vi "Motion Profile Generator-Demo.vi"(0 "Max Speed (rotations/sec)":dbl=3.0, 5 "Max Acceleration (rotations/sec^2)":dbl=1.0, 7 "Max Jerk (rotations/sec^3)":dbl=1.0, 9 "Rotations to Travel":dbl=4.0, 11 "Duration MS":dbl=10.0) -> (4 "Position rotations":dbl[](array[numeric]), 6 "velocity rotations/sec":dbl[](array[numeric]), 8 "acceleration rotations/sec^2":dbl[](array[numeric]), 10 "XY Graph":cluster{dbl[], dbl[]}[](graph))   [LabVIEW 2015]
panel:
  out "Final Position":dbl
  # "This VI uses the \"Copioli\" Method of Motion Profiling. For more information read this chief delphi thread: http://www.chiefdelphi.com/forums/showthread.php?t=98358&highlight=motion+profile"
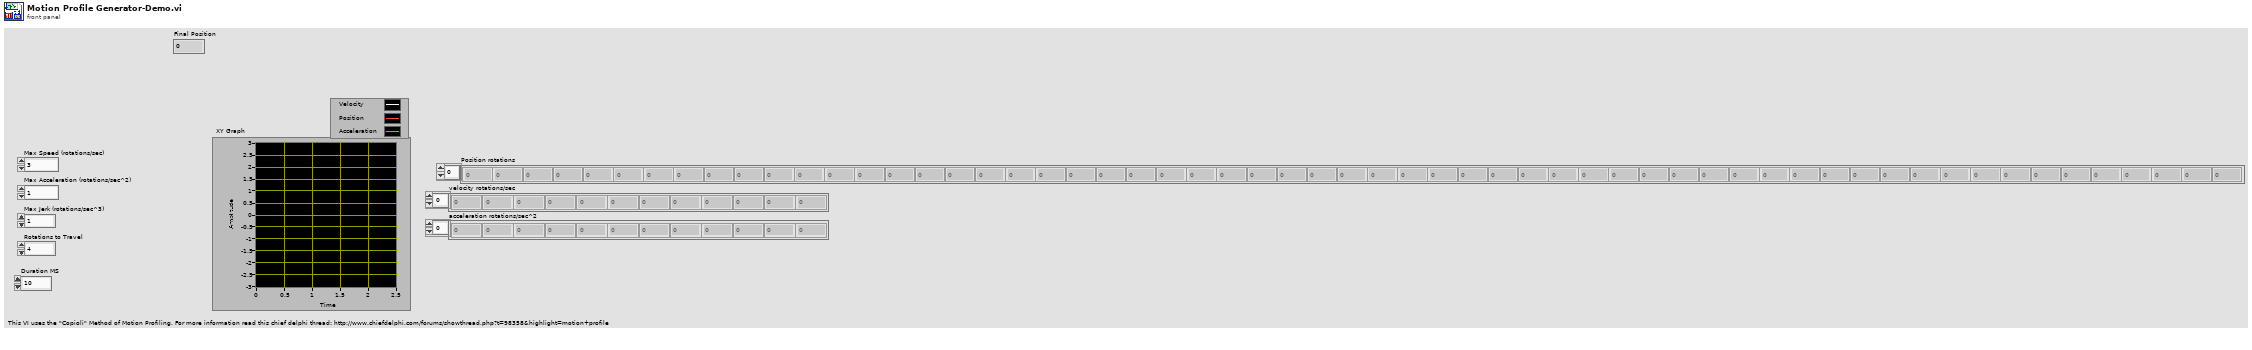
[diagram p1: front panel]
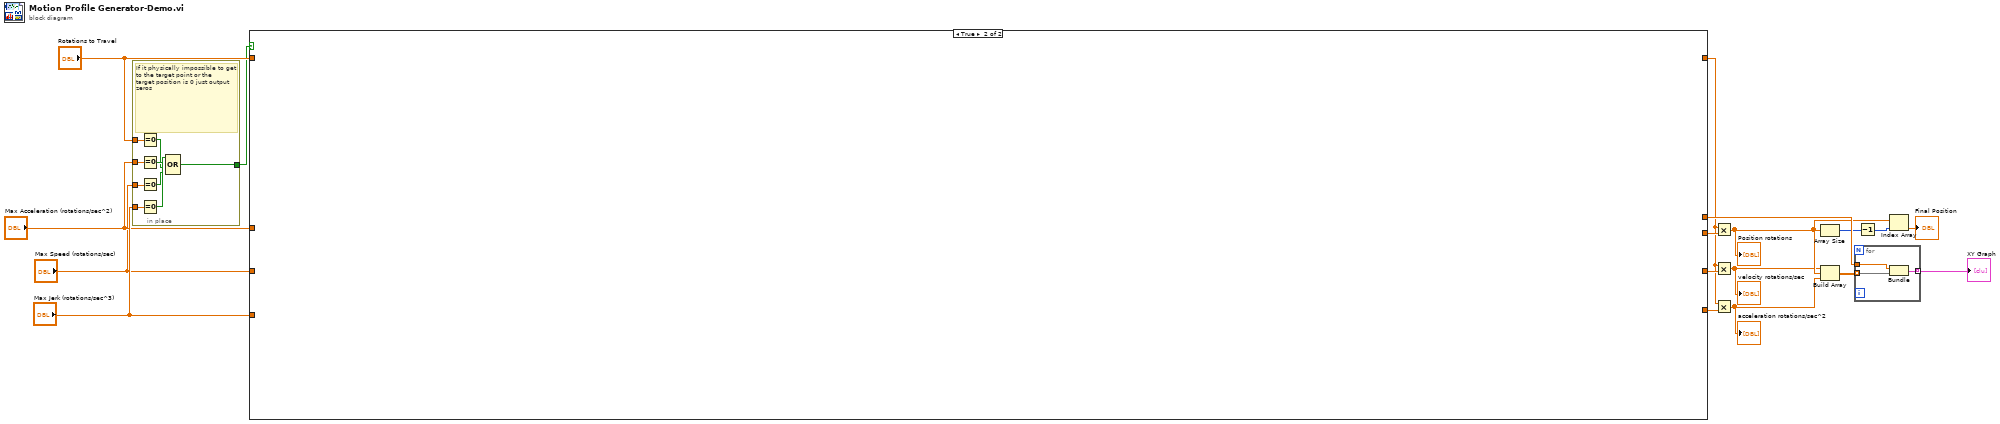
[diagram p0: block diagram]
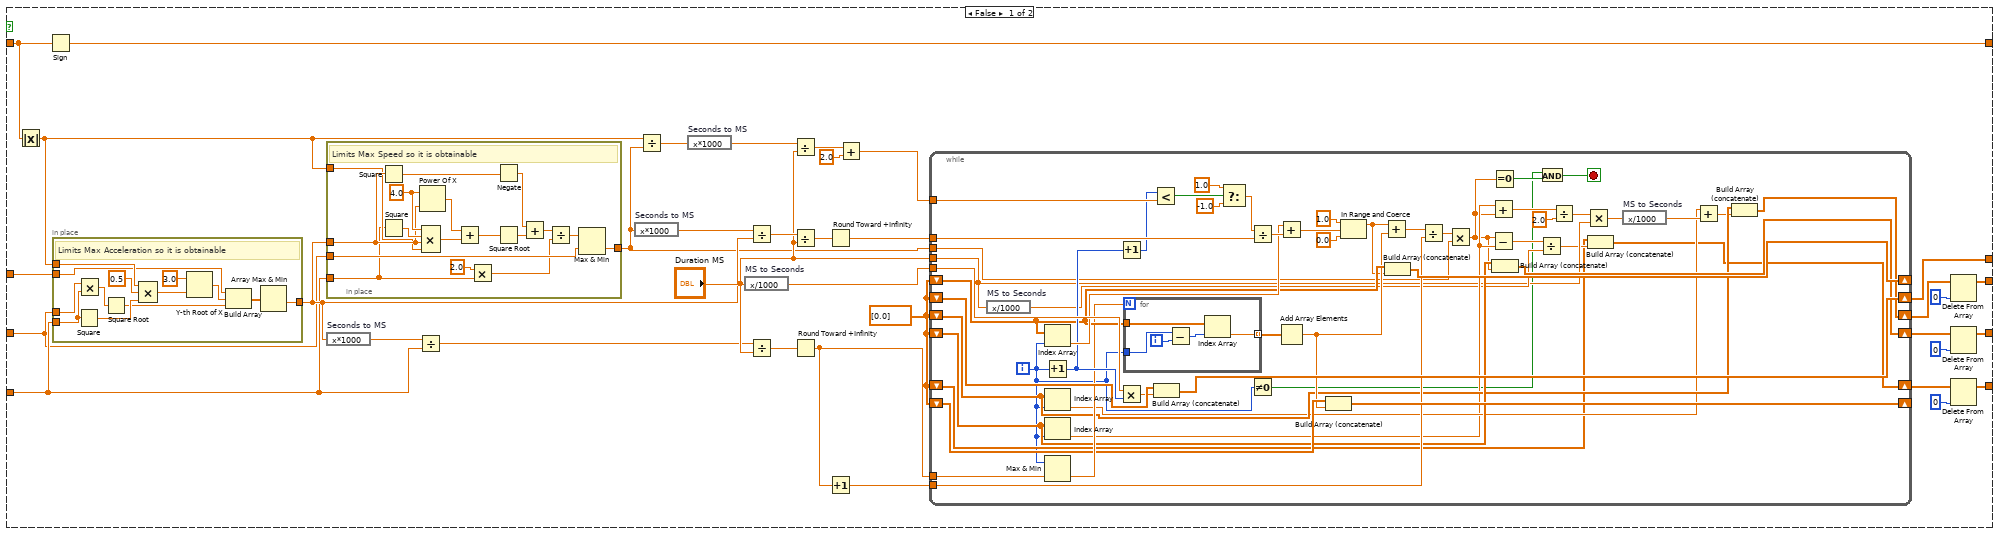
[diagram p2: hidden frame]
diagram:
  n1 = in-place {
    in-place-border: "Max Jerk (rotations/sec^3)" -> [w27]
    in-place-border: "Max Acceleration (rotations/sec^2)" -> [w26]
    in-place-border: "Rotations to Travel" -> [w25]
    in-place-border: [w21] -> w6
    in-place-border: "Max Speed (rotations/sec)" -> [w19]
    # "If it physically impossible to get to the target point or the   target position is 0 just output zeros"
    n2 = Equal To 0?(x=w25) -> (x = 0?=w22:bool)
    n3 = Equal To 0?(x=w26) -> (x = 0?=w23:bool)
    n4 = Equal To 0?(x=w19) -> (x = 0?=w20:bool)
    n5 = Equal To 0?(x=w27) -> (x = 0?=w24:bool)
    n6 = Compound Arithmetic op=OR(w24, w23, w22, w20) -> (w21:bool)
  }
  n7 = case shown="True" w6 {
    tunnel: [w46 _] -> w17
    tunnel: [w40 _] -> w12
    tunnel: [w36 _] -> w11
    tunnel: [w35 _] -> w10
    tunnel: "Max Jerk (rotations/sec^3)" -> [w34 _]
    tunnel: "Max Acceleration (rotations/sec^2)" -> [w33 _]
    tunnel: "Rotations to Travel" -> [w29 _]
    tunnel: "Max Speed (rotations/sec)" -> [w31 _]
    tunnel: [w28 _] -> w1
    frame False {
      w47 = dbl[] [0.0]
      n8 = Absolute Value(x=w29) -> (abs(x)=w30:dbl)
      n9 = Sign(1:w29) -> (0:w28:dbl)
      n10 = in-place {
        in-place-border: w34 -> [w66]
        in-place-border: w33 -> [w70]
        in-place-border: [w63] -> w45
        in-place-border: w30 -> [w75]
        in-place-border: w31 -> [w67]
        # "Limits Max Acceleration so it is obtainable"
        n11 = Square(x=w66) -> (x^2=w73:dbl)
        n12 = Multiply(x=w67, y=w66) -> (x*y=w68:dbl)
        n13 = Square Root(x=w68) -> (sqrt(x)=w65:dbl)
        n14 = Compound Arithmetic op=MULTIPLY(w75, 0.5 ("value"), w73) -> (w72:dbl)
        n15 = Y-th Root of X(1:w72, 2:3.0 ("y")) -> (0:w69:dbl)
        n16 = Build Array(w70, w69, w65) -> (w64:dbl[])
        n17 = Array Max & Min(array=w64) -> (min value=w63:dbl)  [unwired: 3 out]
      }
      n18 = in-place {
        in-place-border: w31 -> [w92]
        in-place-border: [w79] -> w44
        in-place-border: w45 -> [w85]
        in-place-border: w30 -> [w84]
        in-place-border: w34 -> [w81]
        w88 = 4.0 ("x")
        # "Limits Max Speed so it is obtainable"
        n19 = Square(x=w85) -> (x^2=w91:dbl)
        n20 = Square(x=w81) -> (x^2=w87:dbl)
        n21 = Power Of X(1:w85, 2:w88) -> (0:w89:dbl)
        n22 = Compound Arithmetic op=MULTIPLY(w88, w87, w85, w84) -> (w86:dbl)
        n23 = Add(x=w89, y=w86) -> (x+y=w83:dbl)
        n24 = Multiply(x=2.0, y=w81) -> (x*y=w76:dbl)
        n25 = Negate(x=w91) -> (-x=w90:dbl)
        n26 = Square Root(x=w83) -> (sqrt(x)=w80:dbl)
        n27 = Add(x=w90, y=w80) -> (x+y=w78:dbl)
        n28 = Divide(x=w78, y=w76) -> (x/y=w77:dbl)
        n29 = Max & Min(x=w77, y=w92) -> (min(x,y)=w79:dbl)  [unwired: 1 out]
      }
      n30 = expression code="x*1000" "Seconds to MS"(w45) -> (w61:dbl)
      n31 = Divide(x=w61, y=w34) -> (x/y=w32:dbl)
      n32 = expression code="x*1000" "Seconds to MS"(w44) -> (w60:dbl)
      n33 = Divide(x=w30, y=w44) -> (x/y=w59:dbl)
      n34 = expression code="x*1000" "Seconds to MS"(w59) -> (w58:dbl)
      n35 = expression code="x/1000" "MS to Seconds"("Duration MS") -> (w62:dbl)
      n36 = Divide(x=w60, y=w45) -> (x/y=w54:dbl)
      n37 = Divide(x=w32, y="Duration MS") -> (x/y=w51:dbl)
      n38 = Divide(x=w58, y="Duration MS") -> (x/y=w57:dbl)
      n39 = Divide(x=w54, y="Duration MS") -> (x/y=w53:dbl)
      n40 = Round Toward +Infinity(x=w51) -> (ceil(x): smallest int >= x=w50:dbl)
      n41 = Round Toward +Infinity(x=w53) -> (ceil(x): smallest int >= x=w52:dbl)
      n42 = Increment(x=w50) -> (x+1=w49:dbl)
      n43 = Add(x=w57, y=2.0) -> (x+y=w55:dbl)
      n44 = while {
        shift-right: [w144] -> w46
        shift-left: w47 -> [w145]
        tunnel: w62 -> [w143]
        tunnel: w55 -> [w141]
        shift-right: [w131] -> _
        shift-left: w47 -> [w130]
        tunnel: w52 -> [w136]
        tunnel: w50 -> [w128]
        shift-right: [w125] -> _
        shift-left: w47 -> [w126]
        tunnel: w49 -> [w122]
        tunnel: w44 -> [w120]
        shift-right: [w119] -> w39
        shift-left: w47 -> [w117]
        shift-right: [w118] -> w37
        shift-left: w47 -> [w111]
        tunnel: "Duration MS" -> [w105]
        shift-right: [w103] -> w41
        shift-left: w47 -> [w102]
        i -> [w101]
        stop <- w97 stop-if-true
        n45 = expression code="x/1000" "MS to Seconds"(w105) -> (w106:dbl)
        n46 = Index Array(array=w130, index=w101) -> (element=w134:dbl)
        n47 = Increment(x=w101) -> (x+1=w132:i32)
        n48 = Index Array(array=w111, index=w101) -> (element=w110:dbl)
        n49 = Index Array(array=w117, index=w101) -> (element=w108:dbl)
        n50 = Max & Min(x=w101, y=w128) -> (min(x,y)=w127:dbl)  [unwired: 1 out]
        n51 = Increment(x=w132) -> (x+1=w133:i32)
        n52 = Multiply(x=w143, y=w132) -> (x*y=w142:dbl)
        n53 = for {
          N: w127 -> [_]
          tunnel: w101 -> [w149]
          tunnel: w130 -> [w147]
          tunnel: [w146] -> w129 mode=indexing
          i -> [w150]
          n54 = Subtract(x=w149, y=w150) -> (x-y=w148:i32)
          n55 = Index Array(array=w147, index=w148) -> (element=w146:dbl)
        }
        n56 = Less?(x=w133, y=w141) -> (x < y?=w140:bool)
        n57 = Build Array (concatenate)(w145, w142) -> (w144:dbl[])
        n58 = Select(t=1.0, s=w140, f=-1.0) -> (s? t:f=w137:dbl)
        n59 = Divide(x=w137, y=w136) -> (x/y=w135:dbl)
        n60 = Not Equal To 0?(x=w101) -> (x != 0?=w98:bool)
        n61 = Add(x=w134, y=w135) -> (x+y=w94:dbl)
        n62 = Add Array Elements(numeric array=w129) -> (sum=w124:dbl)
        n63 = Build Array (concatenate)(w126, w124) -> (w125:dbl[])
        n64 = In Range and Coerce(upper limit=1.0, x=w94, lower limit=0.0) -> (coerced(x)=w93:dbl)  [unwired: 1 out]
        n65 = Add(x=w93, y=w124) -> (x+y=w123:dbl)
        n66 = Build Array (concatenate)(w130, w93) -> (w131:dbl[])
        n67 = Divide(x=w123, y=w122) -> (x/y=w121:dbl)
        n68 = Multiply(x=w121, y=w120) -> (x*y=w100:dbl)
        n69 = Add(x=w108, y=w100) -> (x+y=w116:dbl)
        n70 = Subtract(x=w100, y=w108) -> (x-y=w107:dbl)
        n71 = Equal To 0?(x=w100) -> (x = 0?=w99:bool)
        n72 = Build Array (concatenate)(w117, w100) -> (w119:dbl[])
        n73 = Divide(x=w107, y=w106) -> (x/y=w104:dbl)
        n74 = And(x=w98, y=w99) -> (x .and. y?=w97:bool)
        n75 = Divide(x=w116, y=2.0) -> (x/y=w114:dbl)
        n76 = Multiply(x=w114, y=w105) -> (x*y=w113:dbl)
        n77 = Build Array (concatenate)(w102, w104) -> (w103:dbl[])
        n78 = expression code="x/1000" "MS to Seconds"(w113) -> (w112:dbl)
        n79 = Add(x=w110, y=w112) -> (x+y=w109:dbl)
        n80 = Build Array (concatenate)(w111, w109) -> (w118:dbl[])
      }
      n81 = Delete From Array(array=w37, index=0) -> (array with subset deleted=w36:dbl[])  [unwired: 1 in, 1 out]
      n82 = Delete From Array(array=w39, index=0) -> (array with subset deleted=w35:dbl[])  [unwired: 1 in, 1 out]
      n83 = Delete From Array(array=w41, index=0) -> (array with subset deleted=w40:dbl[])  [unwired: 1 in, 1 out]
    }
    frame True {
    }
  }
  n84 = Multiply(x=w1, y=w11) -> (x*y=w4:dbl[])
  "Position rotations" <- w4
  n85 = Multiply(x=w1, y=w10) -> (x*y=w3:dbl[])
  "velocity rotations/sec" <- w3
  n86 = Multiply(x=w1, y=w12) -> (x*y=w2:dbl[])
  "acceleration rotations/sec^2" <- w2
  n87 = Array Size(array=w4) -> (size(s)=w15:i32)
  n88 = Build Array(w3, w4, w2) -> (w18:dbl[][])
  n89 = for {
    tunnel: w18 -> [w153] mode=indexing
    tunnel: w17 -> [w152]
    tunnel: [w151] -> w16 mode=indexing
    n90 = Bundle(w152, w153) -> (w151:cluster{dbl[], dbl[]})  [unwired: 1 in]
  }
  "XY Graph" <- w16
  n91 = Decrement(x=w15) -> (x-1=w14:i32)
  n92 = Index Array(array=w4, index=w14) -> (element=→"Final Position":dbl)
